vi "main.vi"() -> ()   [LabVIEW 2025]
uses:
  Global Variable.vi
panel:
  out "catch mouse":picture
  out "2D Picture":picture
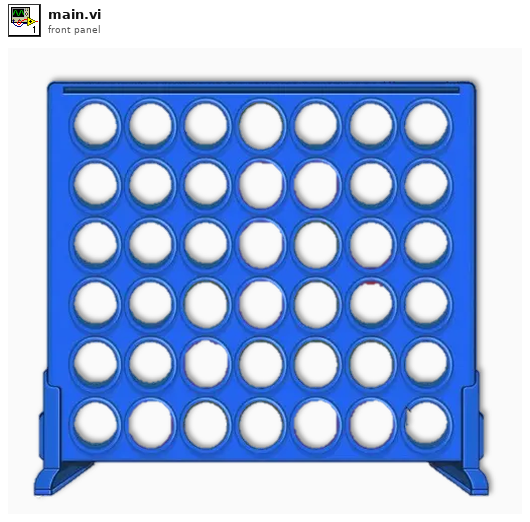
[diagram p1: front panel]
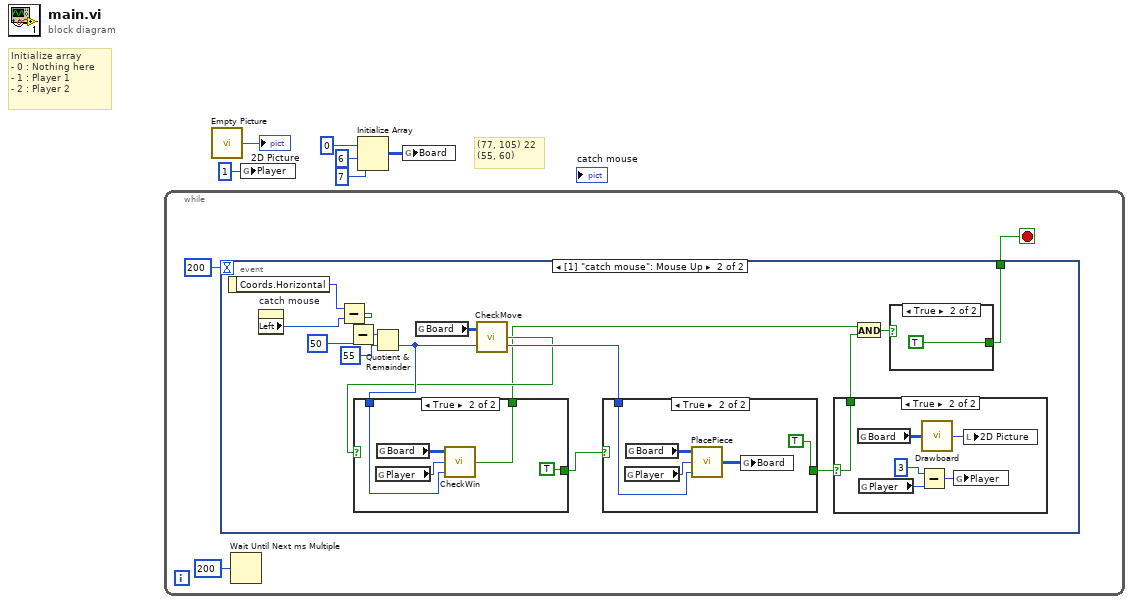
[diagram p0: block diagram]
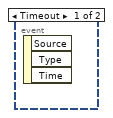
[diagram p2: hidden frame]
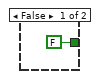
[diagram p3: hidden frame]
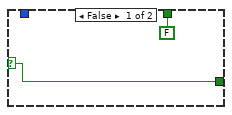
[diagram p4: hidden frame]
diagram:
  # "(77, 105) 22\n(55, 60)"
  # "Initialize array\n- 0 : Nothing here\n- 1 : Player 1\n- 2 : Player 2"
  n1 = while {
    stop <- w7 stop-if-true
    n2 = event shown="[1] \"catch mouse\": Mouse Up" {
      selector: _ -> [_ _]
      dyn-events: _ -> [_ _]
      timeout: 200 -> [_ _]
      tunnel: [_ w10] -> w7
      event Timeout {
        n3 = event-data() -> ()  [unwired: 1 in, 3 out]
      }
      event "catch mouse": Mouse Up {
        n4 = event-data() -> ("Coords.Horizontal"=w18:i32)  [unwired: 1 in]
        n5 = property on="catch mouse" class="Pict"() -> ("Left"=w19:i32)  [unwired: 2 in, 2 out]
        n6 = Subtract(x=w18, y=w19) -> (x-y=w17:i32)
        n7 = Subtract(x=w17, y=50) -> (x-y=w23:i32)
        n8 = Quotient & Remainder(x=w23, y=55) -> (floor(x/y)=w16:i32)  [unwired: 1 out]
        n9 = global read "Global Variable.vi" "Board"() -> (w21:i32[][])
        n10 = call "CheckMove.vi"("col"=w16, "Board"=w21) -> ("Valid"=w15:bool)
        n11 = case shown="True" w15 {
          selector: w15 -> [w28 _]
          tunnel: w16 -> [_ w30]
          tunnel: [w28 TRUE] -> w14
          tunnel: [FALSE ("win") w29] -> w11
          frame False {
          }
          frame True {
            n12 = global read "Global Variable.vi" "Player"() -> (w32:i32)
            n13 = global read "Global Variable.vi" "Board"() -> (w31:i32[][])
            n14 = call "CheckWin.vi"("place"=w30, "player"=w32, "Board"=w31) -> ("win"=w29:bool)
          }
        }
        n15 = case shown="True" w14 {
          selector: w14 -> [w34 _]
          tunnel: w16 -> [_ w36]
          tunnel: [w34 TRUE] -> w20
          frame False {
          }
          frame True {
            n16 = global read "Global Variable.vi" "Player"() -> (w37:i32)
            n17 = global read "Global Variable.vi" "Board"() -> (w38:i32[][])
            n18 = call "PlacePiece.vi"("place"=w36, "player"=w37, "Board"=w38) -> ("board_out"=w39:i32[][])
            n19 = global write "Global Variable.vi" "Board"(w39) -> ()
          }
        }
        n20 = case shown="True" w20 {
          selector: w20 -> [w40 w41]
          tunnel: [w40 w41] -> w12
          frame False {
          }
          frame True {
            n21 = global read "Global Variable.vi" "Board"() -> (w46:i32[][])
            n22 = global read "Global Variable.vi" "Player"() -> (w44:i32)
            n23 = Subtract(x=3, y=w44) -> (x-y=w42:i32)
            n24 = call "Drawboard.vi"("Board"=w46) -> ("2D Picture"=w45:picture)
            n25 = global write "Global Variable.vi" "Player"(w42) -> ()
            n26 = local write "2D Picture"(w45) -> ()
          }
        }
        n27 = And(x=w11, y=w12) -> (x .and. y?=w13:bool)
        n28 = case shown="True" w13 {
          tunnel: [FALSE ("stop") TRUE ("stop")] -> w10
          frame False {
          }
          frame True {
          }
        }
      }
    }
    n29 = Wait Until Next ms Multiple(millisecond multiple=u32 200) -> ()  [unwired: 1 out]
  }
  n30 = call "Empty Picture"() -> ("empty picture"=→"2D Picture":picture)
  n31 = global write "Global Variable.vi" "Player"(1 ("Player")) -> ()
  n32 = Initialize Array(0 ("element"), 6 ("dimension size"), 7 ("dimension size")) -> (w3:i32[][])
  n33 = global write "Global Variable.vi" "Board"(w3) -> ()
